vi "ScanAction.vi"(8 "error in (no error)":errorcluster caption="entrée d'erreur (pas d'erreur)", 9 "IndicePoint":i32, 10 "Dir":bool, 11 "AFG3102C In":refnum<class "AFG3102C.lvclass"> caption="DNL_LabVIEW Object in") -> (0 "error out":errorcluster caption="sortie d'erreur", 2 "ScanParsOut":dbl[](array[numeric]), 3 "AFG3102C Out":refnum<class "AFG3102C.lvclass"> caption="DNL_LabVIEW Object out")   [LabVIEW 2019, in "AFG3102C.lvclass"]
uses:
  AFG3102C.lvclass
  <userlib>/GenProg/ReadValByRefDbl.vi
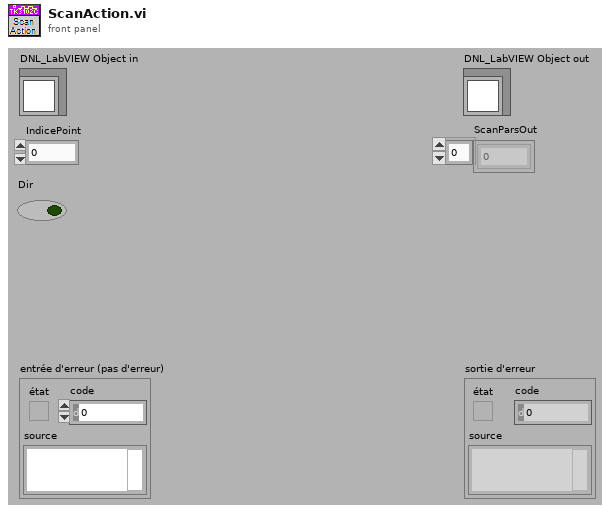
[diagram p1: front panel]
types:
  T1 = typedef "AFG3102C.lvclass/AFG3102C_Func.ctl" = enum16{"Rabi (Tau)", "Ramsey (Tau)"}
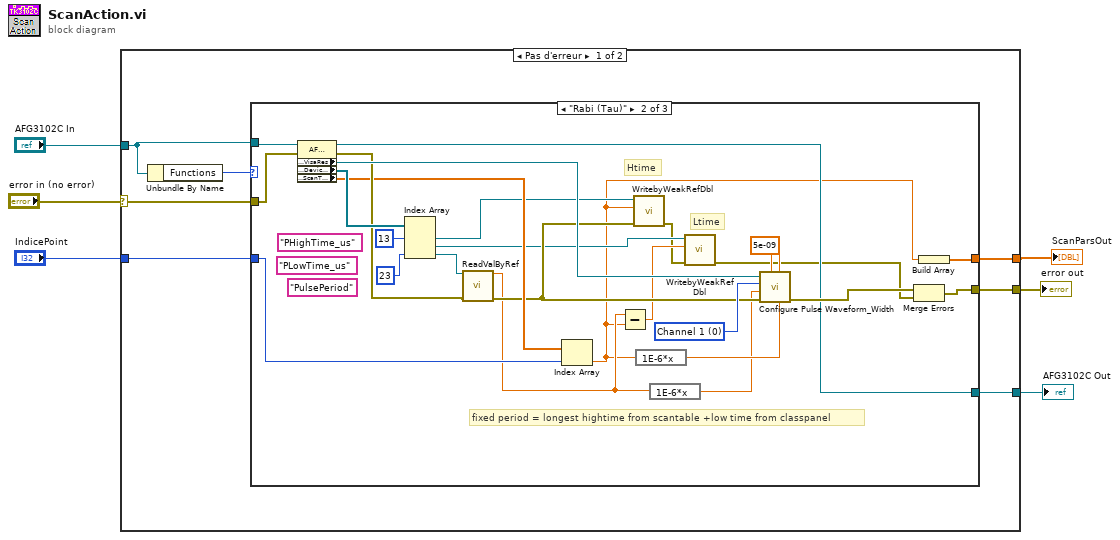
[diagram p0: block diagram]
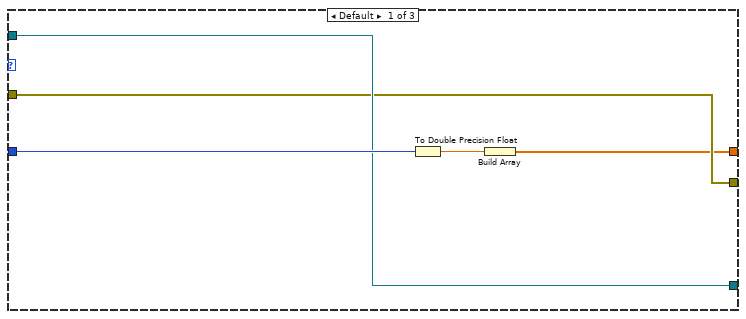
[diagram p2: hidden frame]
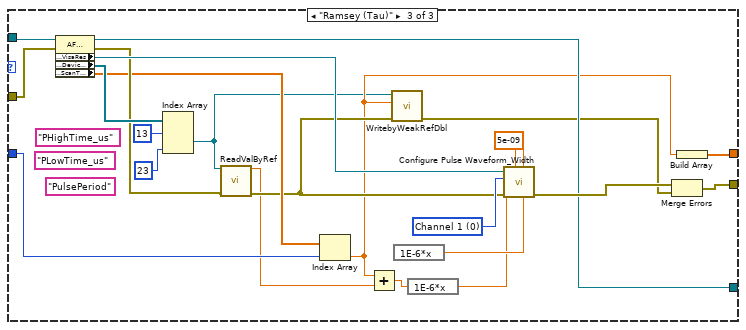
[diagram p3: hidden frame]
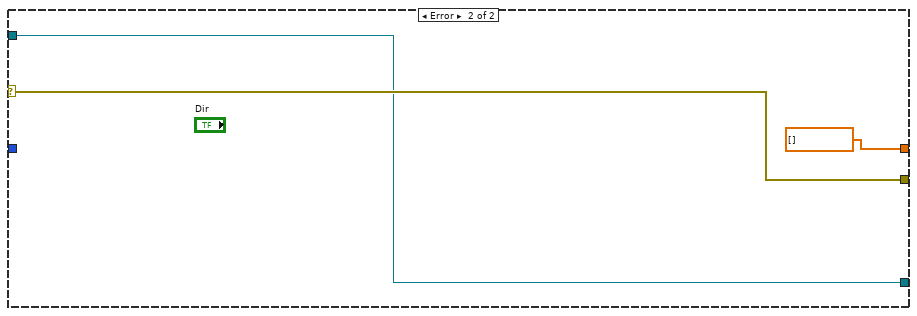
[diagram p4: hidden frame]
diagram:
  n1 = case shown="Pas d'erreur" "error in (no error)" {
    selector: "error in (no error)" -> [w10 w70]
    tunnel: "AFG3102C In" -> [w11 w69]
    tunnel: [w9 dbl[] []] -> w1
    tunnel: [w8 w70] -> w4
    tunnel: [w7 w69] -> w3
    tunnel: "IndicePoint" -> [w12 _]
    frame No Error {
      n2 = Unbundle By Name(w11) -> ("Functions"=w13:T1)
      n3 = case shown="\"Rabi (Tau)\"" w13 {
        tunnel: [w14 w29 w51] -> w9
        tunnel: w12 -> [w18 w32 w55]
        tunnel: [w16 w35 w58] -> w7
        tunnel: w11 -> [w16 w43 w66]
        tunnel: w10 -> [w15 w44 w67]
        tunnel: [w15 w30 w53] -> w8
        frame Default {
          n4 = To Double Precision Float(number=w18) -> (double precision float=w17:dbl)
          n5 = Build Array(w17) -> (w14:dbl[])
        }
        frame "Rabi (Tau)" {
          (unwired) "PulsePeriod" ("ControlName")
          (unwired) "PHighTime_us" ("ControlName")
          (unwired) "PLowTime_us" ("ControlName")
          w42 = 5e-09 ("Leading Edge Time (5.0E-8)")
          w41 = u16 0 items=["Channel 1", "Channel2"] ("Channel (0: Channel 1)")
          # "fixed period = longest hightime from scantable +low time from classpanel"
          # "Ltime"
          # "Htime"
          n6 = property class="AFG3102C.lvclass"(reference=w43, error in=w44) -> (reference out=w35:refnum<class "AFG3102C.lvclass">, error out=w34:errorcluster, "Accessor:VisaRes"=w39:refnum<visa-resource-name>, "Accessor:DeviceCtrl"=w38:refnum<vi>[], "Accessor:ScanTable"=w33:dbl[])
          n7 = Index Array(array=w38, index #1=13 ("indice"), index #3=23 ("indice")) -> (element #1=w25:refnum<vi>, element #2=w24:refnum<vi>, element #3=w26:refnum<vi>)  [unwired: 1 in]
          n8 = call-poly <userlib>:"ReadValByRef.vi"("Control Ref"=w26, "error in"=w34) -> ("Valeur"=w23:dbl, "error out"=w31:errorcluster)  [unwired: 12 in]
          n9 = Index Array(array=w33, index=w32) -> (element=w19:dbl)
          n10 = Subtract(x=w23, y=w19) -> (x-y=w22:dbl)
          n11 = call <userlib>:"WritebyWeakRefDbl.vi"("error in"=w31, "Valeur"=w19, "Control Ref"=w25) -> ("error out"=w21:errorcluster)  [unwired: 8 in]
          n12 = expression code="1E-6*x"(w19) -> (w40:dbl)
          n13 = expression code="1E-6*x"(w23) -> (w28:dbl)
          n14 = call <userlib>:"WritebyWeakRefDbl.vi"("error in"=w21, "Valeur"=w22, "Control Ref"=w24) -> ("error out"=w20:errorcluster)  [unwired: 8 in]
          n15 = call <userlib>:"Configure Pulse Waveform_Width.vi"("Width(s)"=w40, "Trailing Edge Time (5.0E-8)"=w42, "Leading Edge Time (5.0E-8)"=w42, "error in (no error)"=w31, "Period(s)"=w28, "Channel (0: Channel 1)"=w41, "VISA resource name"=w39) -> ("error out"=w36:errorcluster)  [unwired: 3 in, 1 out]
          n16 = Merge Errors(w36, w20) -> (w30:errorcluster)
          n17 = Build Array(w19) -> (w29:dbl[])
        }
        frame "Ramsey (Tau)" {
          (unwired) "PulsePeriod" ("ControlName")
          (unwired) "PHighTime_us" ("ControlName")
          (unwired) "PLowTime_us" ("ControlName")
          w65 = 5e-09 ("Leading Edge Time (5.0E-8)")
          w64 = u16 0 items=["Channel 1", "Channel2"] ("Channel (0: Channel 1)")
          n18 = property class="AFG3102C.lvclass"(reference=w66, error in=w67) -> (reference out=w58:refnum<class "AFG3102C.lvclass">, error out=w57:errorcluster, "Accessor:VisaRes"=w62:refnum<visa-resource-name>, "Accessor:DeviceCtrl"=w61:refnum<vi>[], "Accessor:ScanTable"=w56:dbl[])
          n19 = Index Array(array=w61, index #1=13 ("indice"), index #3=23 ("indice")) -> (element #2=w45:refnum<vi>)  [unwired: 1 in, 2 out]
          n20 = call-poly <userlib>:"ReadValByRef.vi"("Control Ref"=w45, "error in"=w57) -> ("Valeur"=w47:dbl, "error out"=w54:errorcluster)  [unwired: 12 in]
          n21 = Index Array(array=w56, index=w55) -> (element=w48:dbl)
          n22 = Add(x=w48, y=w47) -> (x+y=w46:dbl)
          n23 = call <userlib>:"WritebyWeakRefDbl.vi"("error in"=w54, "Valeur"=w48, "Control Ref"=w45) -> ("error out"=w52:errorcluster)  [unwired: 8 in]
          n24 = expression code="1E-6*x"() -> (w63:dbl)  [unwired: 1 in]
          n25 = expression code="1E-6*x"(w46) -> (w50:dbl)
          n26 = call <userlib>:"Configure Pulse Waveform_Width.vi"("Width(s)"=w63, "Trailing Edge Time (5.0E-8)"=w65, "Leading Edge Time (5.0E-8)"=w65, "error in (no error)"=w54, "Period(s)"=w50, "Channel (0: Channel 1)"=w64, "VISA resource name"=w62) -> ("error out"=w59:errorcluster)  [unwired: 3 in, 1 out]
          n27 = Merge Errors(w59, w52) -> (w53:errorcluster)
          n28 = Build Array(w48) -> (w51:dbl[])
        }
      }
    }
    frame Error {
    }
  }
  "error out" <- w4
  "AFG3102C Out" <- w3
  "ScanParsOut" <- w1
